vi "Advanced Blink Stone Result.vi"(11 "Stone":T1) -> (3 "Result Array":T1[](array[typedef]))   [LabVIEW 2024]
uses:
  Cluster_Blink result.ctl
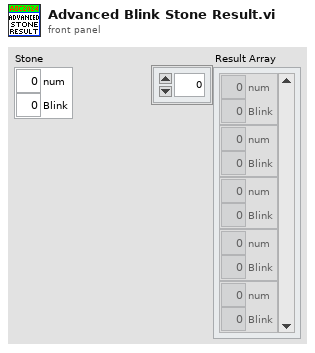
[diagram p1: front panel]
types:
  T1 = typedef "Cluster_Blink result.ctl" = cluster{"num":u64, "Blink":u64}
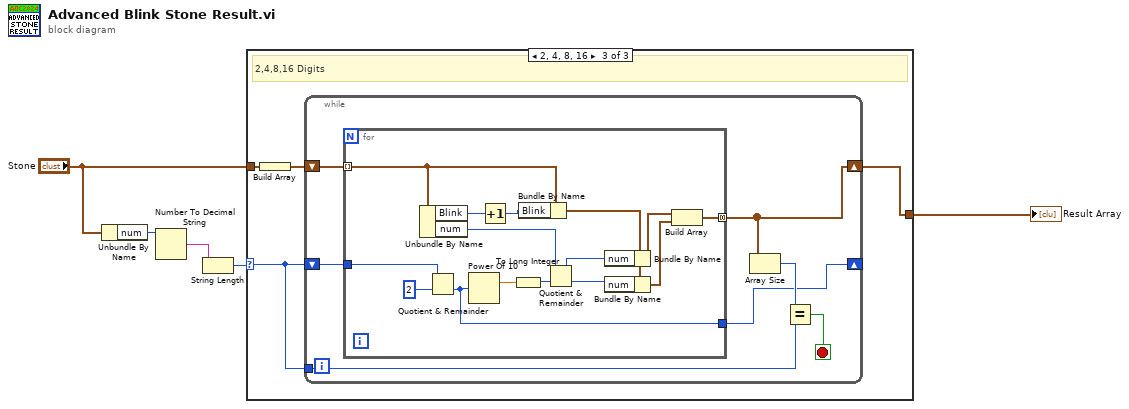
[diagram p0: block diagram]
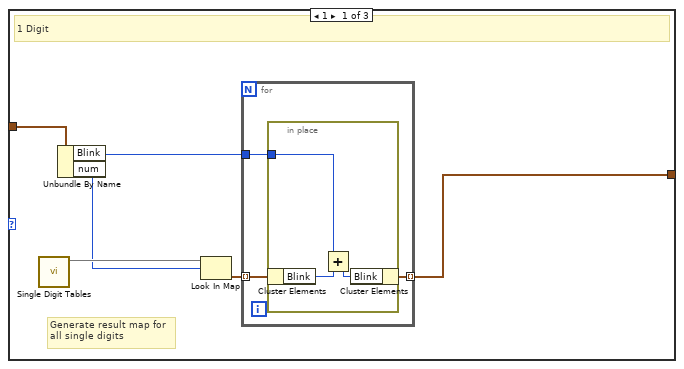
[diagram p2: hidden frame]
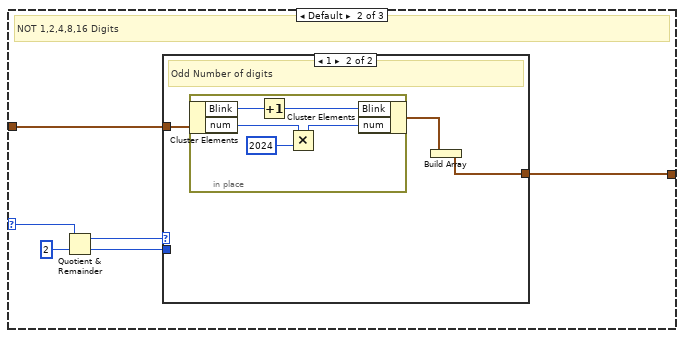
[diagram p3: hidden frame]
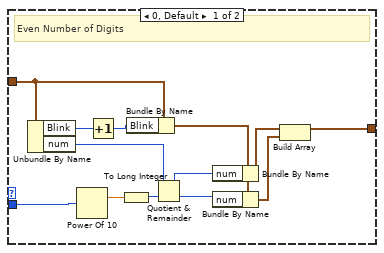
[diagram p4: hidden frame]
diagram:
  n1 = Unbundle By Name("Stone") -> ("num"=w5:u64)
  n2 = Number To Decimal String(number=w5) -> (decimal integer string=w4:string)  [unwired: 1 in]
  n3 = String Length(string=w4) -> (length=w3:i32)
  n4 = case shown="2, 4, 8, 16" w3 {
    selector: w3 -> [_ w20 w45]
    tunnel: [w9 w18 w47] -> w2
    tunnel: "Stone" -> [w8 w19 w48]
    frame 1 {
      # "Generate result map for\nall single digits"
      # "1 Digit"
      n5 = call "Single Digit Tables.vi"() -> ("Map"=w11:map{i32, T1[]})  [unwired: 11 in]
      n6 = Unbundle By Name(w8) -> ("Blink"=w6:u64, "num"=w7:u64)
      n7 = Look In Map(map=w11, key=w7) -> (value=w10:T1[])  [unwired: 1 in, 1 out]
      n8 = for {
        tunnel: w10 -> [w14] mode=indexing
        tunnel: w6 -> [w13]
        tunnel: [w12] -> w9 mode=indexing
        n9 = in-place {
          in-place-border: w13 -> [w15]
          n10 = in-place-cluster #1(w14) -> ("Blink"=w17:u64)
          n11 = Add(x=w15, y=w17) -> (x+y=w16:u64)
          n12 = in-place-cluster #1("Blink"=w16) -> (w12:T1)
        }
      }
    }
    frame Default {
      # "NOT 1,2,4,8,16 Digits"
      n13 = Quotient & Remainder(x=w20, y=2) -> (x-y*floor(x/y)=w23:i32, floor(x/y)=w22:i32)
      n14 = case shown="1" w23 {
        tunnel: w22 -> [w36 _]
        tunnel: [w35 w37] -> w18
        tunnel: w19 -> [w30 w39]
        frame 0, Default {
          # "Even Number of Digits"
          n15 = Unbundle By Name(w30) -> ("Blink"=w31:u64, "num"=w32:u64)
          n16 = Power Of 10(x=w36) -> (10^x=w34:dbl)
          n17 = Increment(x=w31) -> (x+1=w29:u64)
          n18 = To Long Integer(number=w34) -> (32bit integer=w33:i32)
          n19 = Bundle By Name(cluster=w30, "Blink"=w29) -> (w28:T1)
          n20 = Quotient & Remainder(x=w32, y=w33) -> (x-y*floor(x/y)=w27:u64, floor(x/y)=w26:u64)
          n21 = Bundle By Name(cluster=w28, "num"=w27) -> (w25:T1)
          n22 = Bundle By Name(cluster=w28, "num"=w26) -> (w24:T1)
          n23 = Build Array(w25, w24) -> (w35:T1[])
        }
        frame 1 {
          # "Odd Number of digits"
          n24 = in-place {
            n25 = in-place-cluster #2(w39) -> ("Blink"=w43:u64, "num"=w41:u64)
            n26 = Increment(x=w43) -> (x+1=w42:u64)
            n27 = Multiply(x=w41, y=2024) -> (x*y=w40:u64)
            n28 = in-place-cluster #2("Blink"=w42, "num"=w40) -> (w38:T1)
          }
          n29 = Build Array(w38) -> (w37:T1[])
        }
      }
    }
    frame 2, 4, 8, 16 {
      # "2,4,8,16 Digits"
      n30 = Build Array(w48) -> (w46:T1[])
      n31 = while {
        shift-right: [w52] -> w47
        shift-left: w46 -> [w55]
        shift-right: [w49] -> _
        shift-left: w45 -> [w54]
        tunnel: w45 -> [w50]
        stop <- w53 stop-if-true
        n32 = for {
          tunnel: w55 -> [w69] mode=indexing
          tunnel: [w68] -> w52 mode=concatenating
          tunnel: w54 -> [w57]
          tunnel: [w56] -> w49
          n33 = Unbundle By Name(w69) -> ("Blink"=w64:u64, "num"=w65:u64)
          n34 = Quotient & Remainder(x=w57, y=2) -> (floor(x/y)=w56:i32)  [unwired: 1 out]
          n35 = Power Of 10(x=w56) -> (10^x=w67:dbl)
          n36 = Increment(x=w64) -> (x+1=w63:u64)
          n37 = To Long Integer(number=w67) -> (32bit integer=w66:i32)
          n38 = Bundle By Name(cluster=w69, "Blink"=w63) -> (w62:T1)
          n39 = Quotient & Remainder(x=w65, y=w66) -> (x-y*floor(x/y)=w61:u64, floor(x/y)=w60:u64)
          n40 = Bundle By Name(cluster=w62, "num"=w61) -> (w59:T1)
          n41 = Bundle By Name(cluster=w62, "num"=w60) -> (w58:T1)
          n42 = Build Array(w59, w58) -> (w68:T1[])
        }
        n43 = Array Size(array=w52) -> (size(s)=w51:i32)
        n44 = Equal?(x=w51, y=w50) -> (x = y?=w53:bool)
      }
    }
  }
  "Result Array" <- w2
